vi "Write Value.vi"(6 "Gantry in":refnum<class "Gantry.lvclass">, 8 "error in (no error)":errorcluster, 9 "Value":T1, 10 "Address":string, 11 "gScript Interpreter in":refnum<class "gScript Interpreter.lvclass">) -> (0 "error out":errorcluster, 3 "gScript Interpreter out":refnum<class "gScript Interpreter.lvclass">, 4 "Gantry out":refnum<class "Gantry.lvclass">)   [LabVIEW 2026, in "gScript Interpreter.lvclass"]
uses:
  gScript Interpreter.lvclass
  Type Definitions/Memory Cell.ctl
  Type Definitions/Memory Cell Type Enum.ctl
  Shared Components/Gantry Class/Gantry.lvclass
  <vilib>/Utility/error.llb/Error Cluster From Error Code.vi
  <vilib>/ErrorRing/Error Ring.xnode
  Shared Components/FlexWorktable/FlexWorktable.lvclass
  gScript Interpreter.lvclass/gScript Interpreter.ctl
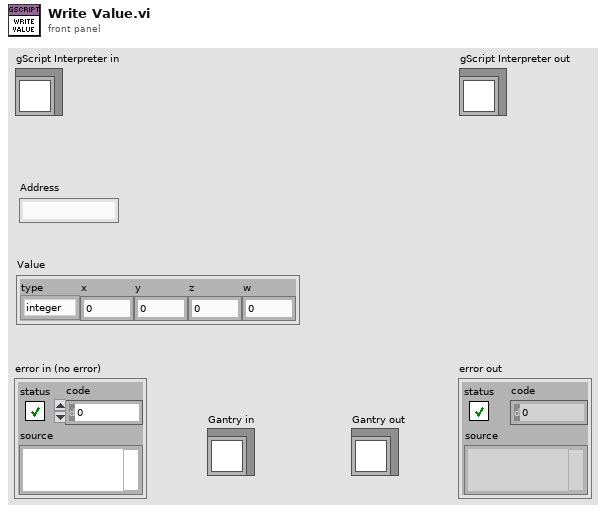
[diagram p1: front panel]
types:
  T1 = typedef "Memory Cell.ctl" = cluster{"type":T2, "x":dbl, "y":dbl, "z":dbl, "w":dbl}
  T2 = typedef "Memory Cell Type Enum.ctl" = enum16{"integer", "float", "vector", "rotation"}
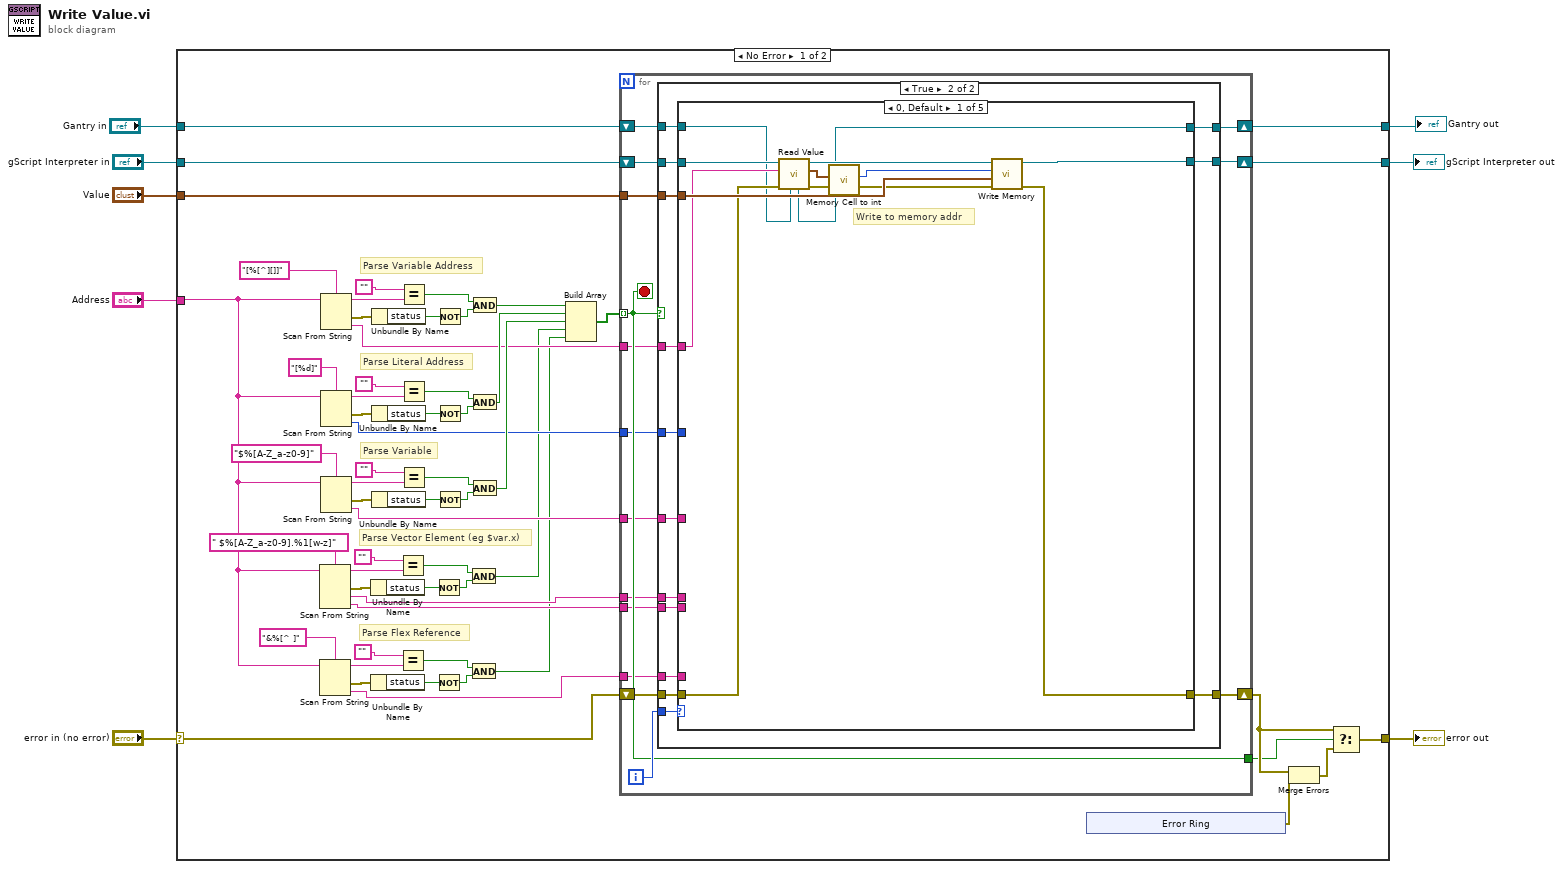
[diagram p0: block diagram]
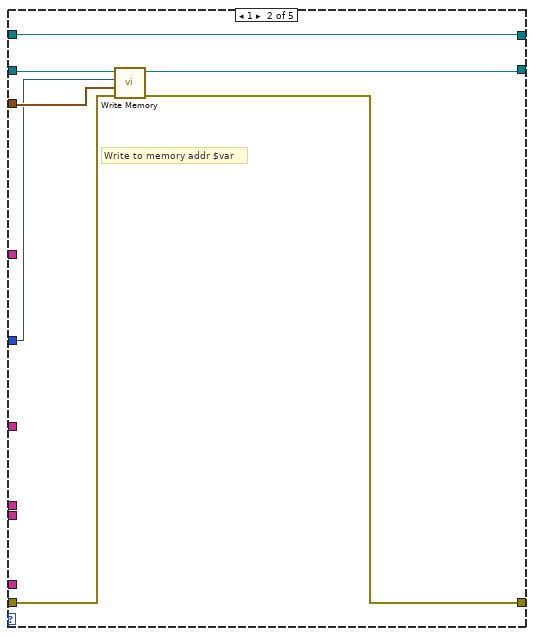
[diagram p3: hidden frame]
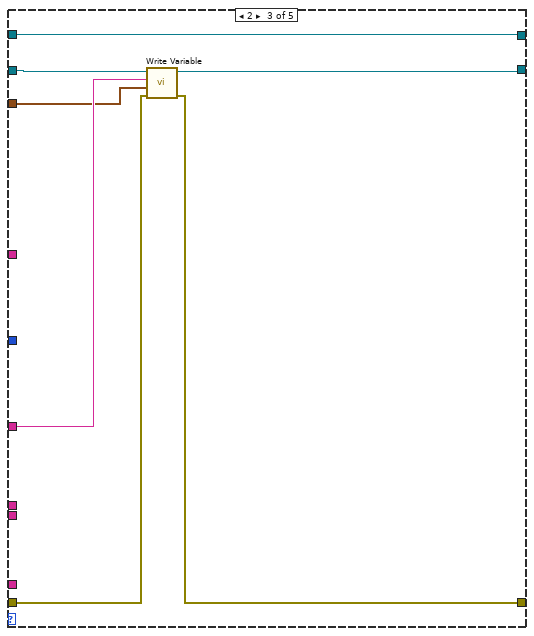
[diagram p4: hidden frame]
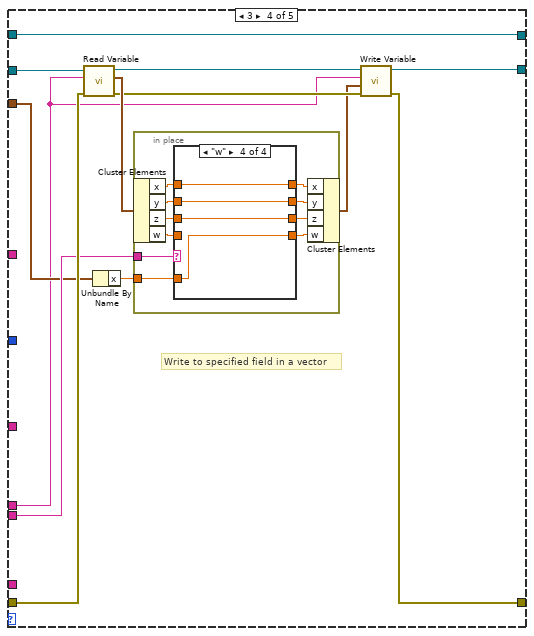
[diagram p5: hidden frame]
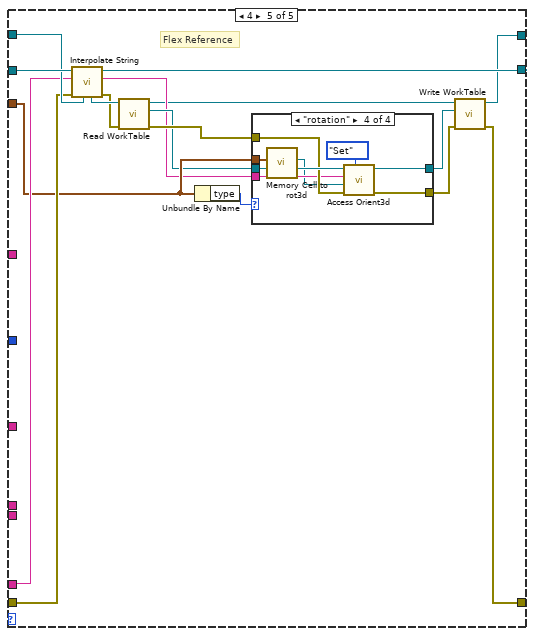
[diagram p9: hidden frame]
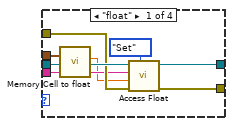
[diagram p10: hidden frame]
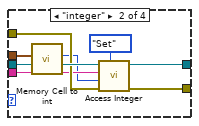
[diagram p11: hidden frame]
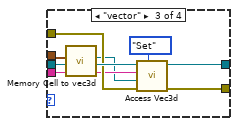
[diagram p12: hidden frame]
diagram:
  n1 = case shown="No Error" "error in (no error)" {
    selector: "error in (no error)" -> [w9 w220]
    tunnel: [w32 w220] -> w7
    tunnel: [w37 w219] -> w5
    tunnel: "gScript Interpreter in" -> [w43 w219]
    tunnel: "Value" -> [w41 _]
    tunnel: "Address" -> [w13 _]
    tunnel: "Gantry in" -> [w21 w218]
    tunnel: [w10 w218] -> w1
    frame No Error {
      # "Parse Flex Reference"
      # "Parse Vector Element (eg $var.x)"
      # "Parse Variable"
      # "Parse Literal Address"
      # "Parse Variable Address"
      n2 = Scan From String(format string=" $%[A-Z_a-z0-9].%1[w-z]", input string=w13) -> (remaining string=w30:string, error out=w28:errorcluster, output 1=w24:string, output 2=w23:string)  [unwired: 4 in, 1 out]
      n3 = Scan From String(format string="&%[^ ]", input string=w13) -> (remaining string=w19:string, error out=w17:errorcluster, output 1=w12:string)  [unwired: 3 in, 1 out]
      n4 = Scan From String(format string="[%[^][]]", input string=w13) -> (remaining string=w66:string, error out=w64:errorcluster, output 1=w40:string)  [unwired: 3 in, 1 out]
      n5 = Scan From String(format string="[%d]", input string=w13) -> (remaining string=w59:string, error out=w57:errorcluster, output 1=w39:i32)  [unwired: 3 in, 1 out]
      n6 = Scan From String(format string="$%[A-Z_a-z0-9]", input string=w13) -> (remaining string=w52:string, error out=w50:errorcluster, output 1=w38:string)  [unwired: 3 in, 1 out]
      n7 = Unbundle By Name(w28) -> ("status"=w26:bool)
      n8 = Unbundle By Name(w17) -> ("status"=w15:bool)
      n9 = Unbundle By Name(w64) -> ("status"=w62:bool)
      n10 = Unbundle By Name(w57) -> ("status"=w55:bool)
      n11 = Unbundle By Name(w50) -> ("status"=w48:bool)
      n12 = Equal?(x="", y=w30) -> (x = y?=w27:bool)
      n13 = Equal?(x="", y=w19) -> (x = y?=w16:bool)
      n14 = Equal?(x="", y=w66) -> (x = y?=w63:bool)
      n15 = Equal?(x="", y=w59) -> (x = y?=w56:bool)
      n16 = Equal?(x="", y=w52) -> (x = y?=w49:bool)
      n17 = Not(x=w26) -> (.not. x?=w25:bool)
      n18 = Not(x=w15) -> (.not. x?=w14:bool)
      n19 = Not(x=w62) -> (.not. x?=w61:bool)
      n20 = Not(x=w55) -> (.not. x?=w54:bool)
      n21 = Not(x=w48) -> (.not. x?=w47:bool)
      n22 = And(x=w27, y=w25) -> (x .and. y?=w22:bool)
      n23 = And(x=w16, y=w14) -> (x .and. y?=w11:bool)
      n24 = And(x=w63, y=w61) -> (x .and. y?=w46:bool)
      n25 = And(x=w56, y=w54) -> (x .and. y?=w45:bool)
      n26 = And(x=w49, y=w47) -> (x .and. y?=w44:bool)
      n27 = Build Array(w46, w45, w44, w22, w11) -> (w42:bool[])
      n28 = for {
        shift-right: [w83] -> w37
        shift-left: w43 -> [w84]
        tunnel: w42 -> [w85] mode=indexing
        tunnel: [w85] -> w33
        tunnel: w41 -> [w82]
        shift-right: [w80] -> w34
        shift-left: w9 -> [w81]
        tunnel: w40 -> [w79]
        tunnel: w39 -> [w78]
        tunnel: w38 -> [w77]
        tunnel: w24 -> [w76]
        tunnel: w23 -> [w75]
        tunnel: w12 -> [w73]
        shift-right: [w72] -> w10
        shift-left: w21 -> [w74]
        i -> [w86]
        stop <- w85 stop-if-true
        n29 = case shown="True" w85 {
          tunnel: w86 -> [_ w103]
          tunnel: w84 -> [w89 w102]
          tunnel: [w89 w101] -> w83
          tunnel: w82 -> [_ w100]
          tunnel: w81 -> [w88 w99]
          tunnel: [w88 w98] -> w80
          tunnel: w79 -> [_ w97]
          tunnel: w78 -> [_ w96]
          tunnel: w77 -> [_ w95]
          tunnel: w76 -> [_ w94]
          tunnel: w75 -> [_ w93]
          tunnel: w74 -> [w87 w92]
          tunnel: w73 -> [_ w91]
          tunnel: [w87 w90] -> w72
          frame False {
          }
          frame True {
            n30 = case shown="0, Default" w103 {
              tunnel: w102 -> [w111 w122 w129 w142 w185]
              tunnel: [w115 w121 w128 w134 w179] -> w101
              tunnel: w100 -> [w113 w120 w124 w138 w178]
              tunnel: w99 -> [w108 w118 w127 w141 w182]
              tunnel: [w112 w117 w126 w133 w169] -> w98
              tunnel: w97 -> [w109 _ _ _ _]
              tunnel: w96 -> [_ w119 _ _ _]
              tunnel: w95 -> [_ _ w125 _ _]
              tunnel: w94 -> [_ _ _ w132 _]
              tunnel: w93 -> [_ _ _ w139 _]
              tunnel: w92 -> [w105 w116 w123 w130 w184]
              tunnel: w91 -> [_ _ _ _ w183]
              tunnel: [w104 w116 w123 w130 w170] -> w90
              frame 0, Default {
                # "Write to memory addr"
                n31 = call-dynamic "Read Value.vi"("Gantry in"=w105, "error in (no error)"=w108, "String in"=w109, "gScript Interpreter in"=w111) -> ("error out"=w107:errorcluster, "Memory Cell"=w106:T1, "gScript Interpreter out"=w110:refnum<class "gScript Interpreter.lvclass">, "Gantry out"=w104:refnum<class "Gantry.lvclass">)  [unwired: 4 in]
                n32 = call "Memory Cell to int.vi"("Memory Cell"=w106) -> ("Int out"=w114:i32)  [unwired: 10 in]
                n33 = call-dynamic "Write Memory.vi"("error in (no error)"=w107, "Memory Cell"=w113, "Memory Address"=w114, "gScript Interpreter in"=w110) -> ("error out"=w112:errorcluster, "gScript Interpreter out"=w115:refnum<class "gScript Interpreter.lvclass">)  [unwired: 6 in]
              }
              frame 1 {
                # "Write to memory addr $var"
                n34 = call-dynamic "Write Memory.vi"("error in (no error)"=w118, "Memory Cell"=w120, "Memory Address"=w119, "gScript Interpreter in"=w122) -> ("error out"=w117:errorcluster, "gScript Interpreter out"=w121:refnum<class "gScript Interpreter.lvclass">)  [unwired: 6 in]
              }
              frame 2 {
                n35 = call-dynamic "Write Variable.vi"("error in (no error)"=w127, "Memory Cell"=w124, "Variable Name"=w125, "gScript Interpreter in"=w129) -> ("error out"=w126:errorcluster, "gScript Interpreter out"=w128:refnum<class "gScript Interpreter.lvclass">)  [unwired: 6 in]
              }
              frame 3 {
                # "Write to specified field in a vector"
                n36 = call-dynamic "Read Variable.vi"("error in (no error)"=w141, "Variable Name"=w132, "gScript Interpreter in"=w142) -> ("error out"=w136:errorcluster, "Memory Cell"=w140:T1, "gScript Interpreter out"=w135:refnum<class "gScript Interpreter.lvclass">)  [unwired: 6 in]
                n37 = Unbundle By Name(w138) -> ("x"=w137:dbl)
                n38 = in-place {
                  in-place-border: w139 -> [w152]
                  in-place-border: w137 -> [w147]
                  n39 = in-place-cluster #1(w140) -> ("x"=w151:dbl, "y"=w150:dbl, "z"=w149:dbl, "w"=w148:dbl)
                  n40 = case shown="\"w\"" w152 {
                    tunnel: w151 -> [_ w159 w163 w167]
                    tunnel: w150 -> [w155 _ w162 w166]
                    tunnel: w149 -> [w154 w158 _ w165]
                    tunnel: w148 -> [w153 w157 w161 _]
                    tunnel: w147 -> [w156 w160 w164 w168]
                    tunnel: [w156 w159 w163 w167] -> w146
                    tunnel: [w155 w160 w162 w166] -> w145
                    tunnel: [w154 w158 w164 w165] -> w144
                    tunnel: [w153 w157 w161 w168] -> w143
                    frame "x", Default {
                    }
                    frame "y" {
                    }
                    frame "z" {
                    }
                    frame "w" {
                    }
                  }
                  n41 = in-place-cluster #1("x"=w146, "y"=w145, "z"=w144, "w"=w143) -> (w131:T1)
                }
                n42 = call-dynamic "Write Variable.vi"("error in (no error)"=w136, "Memory Cell"=w131, "Variable Name"=w132, "gScript Interpreter in"=w135) -> ("error out"=w133:errorcluster, "gScript Interpreter out"=w134:refnum<class "gScript Interpreter.lvclass">)  [unwired: 6 in]
              }
              frame 4 {
                # "Flex Reference"
                n43 = call-dynamic "Interpolate String.vi"("Gantry in"=w184, "error in (no error)"=w182, "Input String"=w183, "gScript Interpreter in"=w185) -> ("error out"=w177:errorcluster, "Output String"=w174:string, "gScript Interpreter out"=w179:refnum<class "gScript Interpreter.lvclass">, "Gantry out"=w181:refnum<class "Gantry.lvclass">)  [unwired: 4 in]
                n44 = call-dynamic "Read WorkTable.vi"("error in"=w177, "Gantry Class in"=w181) -> ("error out"=w176:errorcluster, "Worktable"=w175:refnum<class "FlexWorktable.lvclass">, "Gantry Class out"=w172:refnum<class "Gantry.lvclass">)  [unwired: 7 in]
                n45 = Unbundle By Name(w178) -> ("type"=w180:T2)
                n46 = case shown="\"rotation\"" w180 {
                  tunnel: w175 -> [w193 w201 w209 w217]
                  tunnel: w176 -> [w192 w200 w207 w216]
                  tunnel: [w191 w199 w208 w215] -> w171
                  tunnel: w174 -> [w190 w197 w206 w214]
                  tunnel: w178 -> [w188 w196 w204 w212]
                  tunnel: [w186 w194 w202 w210] -> w173
                  frame "float" {
                    n47 = call "Memory Cell to float.vi"("Memory Cell"=w188) -> ("float out"=w187:dbl)  [unwired: 10 in]
                    n48 = call-dynamic "Access Float.vi"("Get/Set"=enum16{"Get", "Set"}."Set", "error in (no error)"=w192, "Value in"=w187, "Key"=w190, "FlexWorktable in"=w193) -> ("error out"=w191:errorcluster, "FlexWorktable out"=w186:refnum<class "FlexWorktable.lvclass">)  [unwired: 4 in, 1 out]
                  }
                  frame "integer" {
                    n49 = call "Memory Cell to int.vi"("Memory Cell"=w196) -> ("Int out"=w195:i32)  [unwired: 10 in]
                    n50 = call-dynamic "Access Integer.vi"("Get/Set"=enum16{"Get", "Set"}."Set", "error in (no error)"=w200, "Value in"=w195, "Key"=w197, "FlexWorktable in"=w201) -> ("error out"=w199:errorcluster, "FlexWorktable out"=w194:refnum<class "FlexWorktable.lvclass">)  [unwired: 4 in, 1 out]
                  }
                  frame "vector" {
                    n51 = call "Memory Cell to vec3d.vi"("Memory Cell"=w204) -> ("Vec3d out"=w203:refnum<class "Vec3d.lvclass">)  [unwired: 10 in]
                    n52 = call-dynamic "Access Vec3d.vi"("Get/Set"=enum16{"Get", "Set"}."Set", "error in (no error)"=w207, "Value in"=w203, "Key"=w206, "FlexWorktable in"=w209) -> ("error out"=w208:errorcluster, "FlexWorktable out"=w202:refnum<class "FlexWorktable.lvclass">)  [unwired: 4 in, 1 out]
                  }
                  frame "rotation" {
                    n53 = call "Memory Cell to rot3d.vi"("Memory Cell"=w212) -> ("Orient3d out"=w211:refnum<class "Orient3d.lvclass">)  [unwired: 10 in]
                    n54 = call-dynamic "Access Orient3d.vi"("Get/Set"=enum16{"Get", "Set"}."Set", "error in (no error)"=w216, "Value in"=w211, "Key"=w214, "FlexWorktable in"=w217) -> ("error out"=w215:errorcluster, "FlexWorktable out"=w210:refnum<class "FlexWorktable.lvclass">)  [unwired: 4 in, 1 out]
                  }
                }
                n55 = call-dynamic "Write WorkTable.vi"("error in (no error)"=w171, "FlexWorktable"=w173, "Gantry Class in"=w172) -> ("error out"=w169:errorcluster, "Gantry Class out"=w170:refnum<class "Gantry.lvclass">)  [unwired: 7 in]
              }
            }
          }
        }
      }
      n56 = xnode "Error Ring"() -> ("error out"=w36:errorcluster)
      n57 = Merge Errors(w34, w36) -> (w35:errorcluster)
      n58 = Select(t=w34, s=w33, f=w35) -> (s? t:f=w32:errorcluster)
    }
    frame Error {
    }
  }
  "error out" <- w7
  "gScript Interpreter out" <- w5
  "Gantry out" <- w1
